vi "S4GUI.vi"(7 "Tab ObsEng":enum32{"Obs", "CCD modes", "Guider", "Eng"}(tab)) -> ()   [LabVIEW 2018] (continued)
            n4422 = call-dynamic "Write State Machine.vi"("error in (no error)"=w10331, "State Machine.lvclass"=w10334, "Device in"=w10333) -> ("error out"=w10327:errorcluster, "Device out"=w10319:refnum<class "Channel.lvclass">)  [unwired: 7 in]
            n4423 = call-dynamic "Write Channel.vi"("error in (no error)"=w10327, "Channel.lvclass"=w10319, "Acquisition in"=w10332) -> ("error out"=w10328:errorcluster, "Acquisition out"=w10330:refnum<class "Acquisition.lvclass">)  [unwired: 7 in]
            n4424 = call-dynamic "Write AcquisitionC.vi"("error in (no error)"=w10328, "Acquisition.lvclass"=w10330, "S4ACS_GUI in"=w10329) -> ("error out"=w10341:errorcluster, "S4ACS_GUI out"=w10340:refnum<class "S4GUI.lvclass">)  [unwired: 7 in]
          }
        }
      }
      event "cooler ON 4": Value Change {
        n4425 = event-data() -> ("NewVal"=w10342:bool)  [unwired: 1 in]
        n4426 = case shown="True" w10342 {
          tunnel: [w10347 w10382] -> w10346
          tunnel: [w10348 w10381] -> w10345
          tunnel: w10344 -> [w10348 w10352]
          tunnel: w10343 -> [w10347 w10351]
          frame False {
          }
          frame True {
            w10350 = i16 1 items=["Cooler OFF", "Cooler ON"] ("Cooler ON/OFF")
            n4427 = Concatenate Strings("SET COOLER " ("User Event"), "ON ", "CLICKED - CH4" ("User Event")) -> (w10354:string)
            n4428 = call-dynamic "Write User Event.vi"("error in (no error)"=w10351, "User Event"=w10354, "S4GUI in"=w10352) -> ("error out"=w10355:errorcluster, "S4GUI out"=w10357:refnum<class "S4GUI.lvclass">)  [unwired: 7 in]
            n4429 = call-dynamic "Read AcquisitionD.vi"("error in (no error)"=w10355, "S4ACS_GUI in"=w10357) -> ("error out"=w10379:errorcluster, "Acquisition.lvclass"=w10380:refnum<class "Acquisition.lvclass">, "S4ACS_GUI out"=w10370:refnum<class "S4GUI.lvclass">)  [unwired: 7 in]
            n4430 = call-dynamic "Read Channel.vi"("error in (no error)"=w10379, "Acquisition in"=w10380) -> ("error out"=w10363:errorcluster, "Channel.lvclass"=w10367:refnum<class "Channel.lvclass">, "Acquisition out"=w10373:refnum<class "Acquisition.lvclass">)  [unwired: 7 in]
            n4431 = call-dynamic "Read Interface.vi"("error in (no error)"=w10363, "Channel in"=w10367) -> ("error out"=w10358:errorcluster, "Interface.lvclass"=w10359:refnum<class "Interface.lvclass">, "Channel out"=w10366:refnum<class "Channel.lvclass">)  [unwired: 7 in]
            n4432 = call-dynamic "Write Cooler ON_OFF.vi"("error in (no error)"=w10358, "Cooler ON/OFF"=w10350, "Interface in"=w10359) -> ("error out"=w10362:errorcluster, "Interface out"=w10364:refnum<class "Interface.lvclass">)  [unwired: 7 in]
            n4433 = call-dynamic "Write Interface.vi"("error in (no error)"=w10362, "Interface.lvclass"=w10364, "Channel in"=w10366) -> ("error out"=w10361:errorcluster, "Channel out"=w10365:refnum<class "Channel.lvclass">)  [unwired: 7 in]
            n4434 = call-dynamic "Read State Machine.vi"("error in (no error)"=w10361, "Device in"=w10365) -> ("error out"=w10377:errorcluster, "State Machine.lvclass"=w10378:refnum<class "State Machine.lvclass">, "Device out"=w10374:refnum<class "Channel.lvclass">)  [unwired: 7 in]
            n4435 = call "Next State.vi"("error in (no error)"=w10377, "New_State"=u32 30, "State Machine in"=w10378) -> ("error out"=w10372:errorcluster, "State Machine out"=w10375:refnum<class "State Machine.lvclass">)  [unwired: 7 in]
            n4436 = call-dynamic "Write State Machine.vi"("error in (no error)"=w10372, "State Machine.lvclass"=w10375, "Device in"=w10374) -> ("error out"=w10368:errorcluster, "Device out"=w10360:refnum<class "Channel.lvclass">)  [unwired: 7 in]
            n4437 = call-dynamic "Write Channel.vi"("error in (no error)"=w10368, "Channel.lvclass"=w10360, "Acquisition in"=w10373) -> ("error out"=w10369:errorcluster, "Acquisition out"=w10371:refnum<class "Acquisition.lvclass">)  [unwired: 7 in]
            n4438 = call-dynamic "Write AcquisitionD.vi"("error in (no error)"=w10369, "Acquisition.lvclass"=w10371, "S4ACS_GUI in"=w10370) -> ("error out"=w10382:errorcluster, "S4ACS_GUI out"=w10381:refnum<class "S4GUI.lvclass">)  [unwired: 7 in]
          }
        }
      }
      event "cooler OFF 1": Value Change {
        n4439 = event-data() -> ("NewVal"=w10383:bool)  [unwired: 1 in]
        n4440 = case shown="True" w10383 {
          tunnel: [w10388 w10423] -> w10387
          tunnel: [w10389 w10422] -> w10386
          tunnel: w10385 -> [w10389 w10393]
          tunnel: w10384 -> [w10388 w10392]
          frame False {
          }
          frame True {
            w10391 = i16 0 items=["Cooler OFF", "Cooler ON"] ("Cooler ON/OFF")
            n4441 = Concatenate Strings("SET COOLER " ("User Event"), "OFF ", "CLICKED - CH1" ("User Event")) -> (w10395:string)
            n4442 = call-dynamic "Write User Event.vi"("error in (no error)"=w10392, "User Event"=w10395, "S4GUI in"=w10393) -> ("error out"=w10396:errorcluster, "S4GUI out"=w10398:refnum<class "S4GUI.lvclass">)  [unwired: 7 in]
            n4443 = call-dynamic "Read AcquisitionA.vi"("error in (no error)"=w10396, "S4ACS_GUI in"=w10398) -> ("error out"=w10420:errorcluster, "Acquisition.lvclass"=w10421:refnum<class "Acquisition.lvclass">, "S4ACS_GUI out"=w10411:refnum<class "S4GUI.lvclass">)  [unwired: 7 in]
            n4444 = call-dynamic "Read Channel.vi"("error in (no error)"=w10420, "Acquisition in"=w10421) -> ("error out"=w10404:errorcluster, "Channel.lvclass"=w10408:refnum<class "Channel.lvclass">, "Acquisition out"=w10414:refnum<class "Acquisition.lvclass">)  [unwired: 7 in]
            n4445 = call-dynamic "Read Interface.vi"("error in (no error)"=w10404, "Channel in"=w10408) -> ("error out"=w10399:errorcluster, "Interface.lvclass"=w10400:refnum<class "Interface.lvclass">, "Channel out"=w10407:refnum<class "Channel.lvclass">)  [unwired: 7 in]
            n4446 = call-dynamic "Write Cooler ON_OFF.vi"("error in (no error)"=w10399, "Cooler ON/OFF"=w10391, "Interface in"=w10400) -> ("error out"=w10403:errorcluster, "Interface out"=w10405:refnum<class "Interface.lvclass">)  [unwired: 7 in]
            n4447 = call-dynamic "Write Interface.vi"("error in (no error)"=w10403, "Interface.lvclass"=w10405, "Channel in"=w10407) -> ("error out"=w10402:errorcluster, "Channel out"=w10406:refnum<class "Channel.lvclass">)  [unwired: 7 in]
            n4448 = call-dynamic "Read State Machine.vi"("error in (no error)"=w10402, "Device in"=w10406) -> ("error out"=w10418:errorcluster, "State Machine.lvclass"=w10419:refnum<class "State Machine.lvclass">, "Device out"=w10415:refnum<class "Channel.lvclass">)  [unwired: 7 in]
            n4449 = call "Next State.vi"("error in (no error)"=w10418, "New_State"=u32 30, "State Machine in"=w10419) -> ("error out"=w10413:errorcluster, "State Machine out"=w10416:refnum<class "State Machine.lvclass">)  [unwired: 7 in]
            n4450 = call-dynamic "Write State Machine.vi"("error in (no error)"=w10413, "State Machine.lvclass"=w10416, "Device in"=w10415) -> ("error out"=w10409:errorcluster, "Device out"=w10401:refnum<class "Channel.lvclass">)  [unwired: 7 in]
            n4451 = call-dynamic "Write Channel.vi"("error in (no error)"=w10409, "Channel.lvclass"=w10401, "Acquisition in"=w10414) -> ("error out"=w10410:errorcluster, "Acquisition out"=w10412:refnum<class "Acquisition.lvclass">)  [unwired: 7 in]
            n4452 = call-dynamic "Write AcquisitionA.vi"("error in (no error)"=w10410, "Acquisition.lvclass"=w10412, "S4ACS_GUI in"=w10411) -> ("error out"=w10423:errorcluster, "S4ACS_GUI out"=w10422:refnum<class "S4GUI.lvclass">)  [unwired: 7 in]
          }
        }
      }
      event "cooler OFF 2": Value Change {
        n4453 = event-data() -> ("NewVal"=w10424:bool)  [unwired: 1 in]
        n4454 = case shown="True" w10424 {
          tunnel: [w10429 w10464] -> w10428
          tunnel: [w10430 w10463] -> w10427
          tunnel: w10426 -> [w10430 w10434]
          tunnel: w10425 -> [w10429 w10433]
          frame False {
          }
          frame True {
            w10432 = i16 0 items=["Cooler OFF", "Cooler ON"] ("Cooler ON/OFF")
            n4455 = Concatenate Strings("SET COOLER " ("User Event"), "OFF ", "CLICKED - CH2" ("User Event")) -> (w10436:string)
            n4456 = call-dynamic "Write User Event.vi"("error in (no error)"=w10433, "User Event"=w10436, "S4GUI in"=w10434) -> ("error out"=w10437:errorcluster, "S4GUI out"=w10439:refnum<class "S4GUI.lvclass">)  [unwired: 7 in]
            n4457 = call "Read AcquisitionB.vi"("error in (no error)"=w10437, "S4ACS_GUI in"=w10439) -> ("error out"=w10461:errorcluster, "Acquisition.lvclass"=w10462:refnum<class "Acquisition.lvclass">, "S4ACS_GUI out"=w10452:refnum<class "S4GUI.lvclass">)  [unwired: 7 in]
            n4458 = call-dynamic "Read Channel.vi"("error in (no error)"=w10461, "Acquisition in"=w10462) -> ("error out"=w10445:errorcluster, "Channel.lvclass"=w10449:refnum<class "Channel.lvclass">, "Acquisition out"=w10455:refnum<class "Acquisition.lvclass">)  [unwired: 7 in]
            n4459 = call-dynamic "Read Interface.vi"("error in (no error)"=w10445, "Channel in"=w10449) -> ("error out"=w10440:errorcluster, "Interface.lvclass"=w10441:refnum<class "Interface.lvclass">, "Channel out"=w10448:refnum<class "Channel.lvclass">)  [unwired: 7 in]
            n4460 = call-dynamic "Write Cooler ON_OFF.vi"("error in (no error)"=w10440, "Cooler ON/OFF"=w10432, "Interface in"=w10441) -> ("error out"=w10444:errorcluster, "Interface out"=w10446:refnum<class "Interface.lvclass">)  [unwired: 7 in]
            n4461 = call-dynamic "Write Interface.vi"("error in (no error)"=w10444, "Interface.lvclass"=w10446, "Channel in"=w10448) -> ("error out"=w10443:errorcluster, "Channel out"=w10447:refnum<class "Channel.lvclass">)  [unwired: 7 in]
            n4462 = call-dynamic "Read State Machine.vi"("error in (no error)"=w10443, "Device in"=w10447) -> ("error out"=w10459:errorcluster, "State Machine.lvclass"=w10460:refnum<class "State Machine.lvclass">, "Device out"=w10456:refnum<class "Channel.lvclass">)  [unwired: 7 in]
            n4463 = call "Next State.vi"("error in (no error)"=w10459, "New_State"=u32 30, "State Machine in"=w10460) -> ("error out"=w10454:errorcluster, "State Machine out"=w10457:refnum<class "State Machine.lvclass">)  [unwired: 7 in]
            n4464 = call-dynamic "Write State Machine.vi"("error in (no error)"=w10454, "State Machine.lvclass"=w10457, "Device in"=w10456) -> ("error out"=w10450:errorcluster, "Device out"=w10442:refnum<class "Channel.lvclass">)  [unwired: 7 in]
            n4465 = call-dynamic "Write Channel.vi"("error in (no error)"=w10450, "Channel.lvclass"=w10442, "Acquisition in"=w10455) -> ("error out"=w10451:errorcluster, "Acquisition out"=w10453:refnum<class "Acquisition.lvclass">)  [unwired: 7 in]
            n4466 = call "Write AcquisitionB.vi"("error in (no error)"=w10451, "Acquisition.lvclass"=w10453, "S4ACS_GUI in"=w10452) -> ("error out"=w10464:errorcluster, "S4ACS_GUI out"=w10463:refnum<class "S4GUI.lvclass">)  [unwired: 7 in]
          }
        }
      }
      event "cooler OFF 3": Value Change {
        n4467 = event-data() -> ("NewVal"=w10465:bool)  [unwired: 1 in]
        n4468 = case shown="True" w10465 {
          tunnel: [w10470 w10505] -> w10469
          tunnel: [w10471 w10504] -> w10468
          tunnel: w10467 -> [w10471 w10475]
          tunnel: w10466 -> [w10470 w10474]
          frame False {
          }
          frame True {
            w10473 = i16 0 items=["Cooler OFF", "Cooler ON"] ("Cooler ON/OFF")
            n4469 = Concatenate Strings("SET COOLER " ("User Event"), "OFF ", "CLICKED - CH3" ("User Event")) -> (w10477:string)
            n4470 = call-dynamic "Write User Event.vi"("error in (no error)"=w10474, "User Event"=w10477, "S4GUI in"=w10475) -> ("error out"=w10478:errorcluster, "S4GUI out"=w10480:refnum<class "S4GUI.lvclass">)  [unwired: 7 in]
            n4471 = call-dynamic "Read AcquisitionC.vi"("error in (no error)"=w10478, "S4ACS_GUI in"=w10480) -> ("error out"=w10502:errorcluster, "Acquisition.lvclass"=w10503:refnum<class "Acquisition.lvclass">, "S4ACS_GUI out"=w10493:refnum<class "S4GUI.lvclass">)  [unwired: 7 in]
            n4472 = call-dynamic "Read Channel.vi"("error in (no error)"=w10502, "Acquisition in"=w10503) -> ("error out"=w10486:errorcluster, "Channel.lvclass"=w10490:refnum<class "Channel.lvclass">, "Acquisition out"=w10496:refnum<class "Acquisition.lvclass">)  [unwired: 7 in]
            n4473 = call-dynamic "Read Interface.vi"("error in (no error)"=w10486, "Channel in"=w10490) -> ("error out"=w10481:errorcluster, "Interface.lvclass"=w10482:refnum<class "Interface.lvclass">, "Channel out"=w10489:refnum<class "Channel.lvclass">)  [unwired: 7 in]
            n4474 = call-dynamic "Write Cooler ON_OFF.vi"("error in (no error)"=w10481, "Cooler ON/OFF"=w10473, "Interface in"=w10482) -> ("error out"=w10485:errorcluster, "Interface out"=w10487:refnum<class "Interface.lvclass">)  [unwired: 7 in]
            n4475 = call-dynamic "Write Interface.vi"("error in (no error)"=w10485, "Interface.lvclass"=w10487, "Channel in"=w10489) -> ("error out"=w10484:errorcluster, "Channel out"=w10488:refnum<class "Channel.lvclass">)  [unwired: 7 in]
            n4476 = call-dynamic "Read State Machine.vi"("error in (no error)"=w10484, "Device in"=w10488) -> ("error out"=w10500:errorcluster, "State Machine.lvclass"=w10501:refnum<class "State Machine.lvclass">, "Device out"=w10497:refnum<class "Channel.lvclass">)  [unwired: 7 in]
            n4477 = call "Next State.vi"("error in (no error)"=w10500, "New_State"=u32 30, "State Machine in"=w10501) -> ("error out"=w10495:errorcluster, "State Machine out"=w10498:refnum<class "State Machine.lvclass">)  [unwired: 7 in]
            n4478 = call-dynamic "Write State Machine.vi"("error in (no error)"=w10495, "State Machine.lvclass"=w10498, "Device in"=w10497) -> ("error out"=w10491:errorcluster, "Device out"=w10483:refnum<class "Channel.lvclass">)  [unwired: 7 in]
            n4479 = call-dynamic "Write Channel.vi"("error in (no error)"=w10491, "Channel.lvclass"=w10483, "Acquisition in"=w10496) -> ("error out"=w10492:errorcluster, "Acquisition out"=w10494:refnum<class "Acquisition.lvclass">)  [unwired: 7 in]
            n4480 = call-dynamic "Write AcquisitionC.vi"("error in (no error)"=w10492, "Acquisition.lvclass"=w10494, "S4ACS_GUI in"=w10493) -> ("error out"=w10505:errorcluster, "S4ACS_GUI out"=w10504:refnum<class "S4GUI.lvclass">)  [unwired: 7 in]
          }
        }
      }
      event "cooler OFF 4": Value Change {
        n4481 = event-data() -> ("NewVal"=w10506:bool)  [unwired: 1 in]
        n4482 = case shown="True" w10506 {
          tunnel: [w10511 w10546] -> w10510
          tunnel: [w10512 w10545] -> w10509
          tunnel: w10508 -> [w10512 w10516]
          tunnel: w10507 -> [w10511 w10515]
          frame False {
          }
          frame True {
            w10514 = i16 0 items=["Cooler OFF", "Cooler ON"] ("Cooler ON/OFF")
            n4483 = Concatenate Strings("SET COOLER " ("User Event"), "OFF ", "CLICKED - CH4" ("User Event")) -> (w10518:string)
            n4484 = call-dynamic "Write User Event.vi"("error in (no error)"=w10515, "User Event"=w10518, "S4GUI in"=w10516) -> ("error out"=w10519:errorcluster, "S4GUI out"=w10521:refnum<class "S4GUI.lvclass">)  [unwired: 7 in]
            n4485 = call-dynamic "Read AcquisitionD.vi"("error in (no error)"=w10519, "S4ACS_GUI in"=w10521) -> ("error out"=w10543:errorcluster, "Acquisition.lvclass"=w10544:refnum<class "Acquisition.lvclass">, "S4ACS_GUI out"=w10534:refnum<class "S4GUI.lvclass">)  [unwired: 7 in]
            n4486 = call-dynamic "Read Channel.vi"("error in (no error)"=w10543, "Acquisition in"=w10544) -> ("error out"=w10527:errorcluster, "Channel.lvclass"=w10531:refnum<class "Channel.lvclass">, "Acquisition out"=w10537:refnum<class "Acquisition.lvclass">)  [unwired: 7 in]
            n4487 = call-dynamic "Read Interface.vi"("error in (no error)"=w10527, "Channel in"=w10531) -> ("error out"=w10522:errorcluster, "Interface.lvclass"=w10523:refnum<class "Interface.lvclass">, "Channel out"=w10530:refnum<class "Channel.lvclass">)  [unwired: 7 in]
            n4488 = call-dynamic "Write Cooler ON_OFF.vi"("error in (no error)"=w10522, "Cooler ON/OFF"=w10514, "Interface in"=w10523) -> ("error out"=w10526:errorcluster, "Interface out"=w10528:refnum<class "Interface.lvclass">)  [unwired: 7 in]
            n4489 = call-dynamic "Write Interface.vi"("error in (no error)"=w10526, "Interface.lvclass"=w10528, "Channel in"=w10530) -> ("error out"=w10525:errorcluster, "Channel out"=w10529:refnum<class "Channel.lvclass">)  [unwired: 7 in]
            n4490 = call-dynamic "Read State Machine.vi"("error in (no error)"=w10525, "Device in"=w10529) -> ("error out"=w10541:errorcluster, "State Machine.lvclass"=w10542:refnum<class "State Machine.lvclass">, "Device out"=w10538:refnum<class "Channel.lvclass">)  [unwired: 7 in]
            n4491 = call "Next State.vi"("error in (no error)"=w10541, "New_State"=u32 30, "State Machine in"=w10542) -> ("error out"=w10536:errorcluster, "State Machine out"=w10539:refnum<class "State Machine.lvclass">)  [unwired: 7 in]
            n4492 = call-dynamic "Write State Machine.vi"("error in (no error)"=w10536, "State Machine.lvclass"=w10539, "Device in"=w10538) -> ("error out"=w10532:errorcluster, "Device out"=w10524:refnum<class "Channel.lvclass">)  [unwired: 7 in]
            n4493 = call-dynamic "Write Channel.vi"("error in (no error)"=w10532, "Channel.lvclass"=w10524, "Acquisition in"=w10537) -> ("error out"=w10533:errorcluster, "Acquisition out"=w10535:refnum<class "Acquisition.lvclass">)  [unwired: 7 in]
            n4494 = call-dynamic "Write AcquisitionD.vi"("error in (no error)"=w10533, "Acquisition.lvclass"=w10535, "S4ACS_GUI in"=w10534) -> ("error out"=w10546:errorcluster, "S4ACS_GUI out"=w10545:refnum<class "S4GUI.lvclass">)  [unwired: 7 in]
          }
        }
      }
      event "Set Temp 1": Value Change {
        n4495 = event-data() -> ("NewVal"=w10547:bool)  [unwired: 1 in]
        n4496 = case shown="True" w10547 {
          tunnel: w10551 -> [w10553 w10570]
          tunnel: w10550 -> [w10552 w10569]
          tunnel: [w10552 w10559] -> w10549
          tunnel: [w10553 w10560] -> w10548
          frame False {
          }
          frame True {
            # "Carrega a maior temperatura\nentre target atual e o target do controle."
            # "Carrega o valor da temperatura target de acordo com a conf CCD"
            n4497 = call-dynamic "Read AcquisitionA.vi"("error in (no error)"=w10569, "S4ACS_GUI in"=w10570) -> ("error out"=w10572:errorcluster, "Acquisition.lvclass"=w10571:refnum<class "Acquisition.lvclass">, "S4ACS_GUI out"=w10556:refnum<class "S4GUI.lvclass">)  [unwired: 7 in]
            n4498 = call-dynamic "Read Channel.vi"("error in (no error)"=w10572, "Acquisition in"=w10571) -> ("error out"=w10583:errorcluster, "Channel.lvclass"=w10582:refnum<class "Channel.lvclass">, "Acquisition out"=w10555:refnum<class "Acquisition.lvclass">)  [unwired: 7 in]
            n4499 = call-dynamic "ValidateConfig.vi"("error in (no error)"=w10583, "Channel in"=w10582) -> ("error out"=w10589:errorcluster, "Channel out"=w10588:refnum<class "Channel.lvclass">)  [unwired: 7 in, 1 out]
            n4500 = call-dynamic "Read Interface.vi"("error in (no error)"=w10589, "Channel in"=w10588) -> ("error out"=w10585:errorcluster, "Interface.lvclass"=w10584:refnum<class "Interface.lvclass">, "Channel out"=w10578:refnum<class "Channel.lvclass">)  [unwired: 7 in]
            n4501 = call-dynamic "Read Temperature.vi"("error in (no error)"=w10585, "Interface in"=w10584) -> ("error out"=w10586:errorcluster, "Temperature"=w10590:i8, "Interface out"=w10587:refnum<class "Interface.lvclass">)  [unwired: 7 in]
            n4502 = Greater?(x=w10590, y="Target Temp 1") -> (0:w10558:bool)
            n4503 = Select(t=w10590, s=w10558, f="Target Temp 1") -> (s? t:f=w10563:i8)
            n4504 = call-dynamic "Write Temperature.vi"("error in (no error)"=w10586, "Temperature"=w10563, "Interface in"=w10587) -> ("error out"=w10580:errorcluster, "Interface out"=w10577:refnum<class "Interface.lvclass">)  [unwired: 7 in]
            n4505 = call-dynamic "Write Interface.vi"("error in (no error)"=w10580, "Interface.lvclass"=w10577, "Channel in"=w10578) -> ("error out"=w10581:errorcluster, "Channel out"=w10579:refnum<class "Channel.lvclass">)  [unwired: 7 in]
            n4506 = case shown="True" w10558 {
              tunnel: w10581 -> [w10615 w10618]
              tunnel: w10579 -> [w10614 w10625]
              tunnel: [w10613 w10625] -> w10576
              tunnel: [w10612 w10624] -> w10575
              tunnel: w10556 -> [w10592 w10620]
              tunnel: [w10592 w10623] -> w10557
              tunnel: w10555 -> [w10591 w10622]
              tunnel: [w10591 w10621] -> w10554
              frame False {
                # "input ok"
                n4507 = call-dynamic "Read State Machine.vi"("error in (no error)"=w10615, "Device in"=w10614) -> ("error out"=w10594:errorcluster, "State Machine.lvclass"=w10601:refnum<class "State Machine.lvclass">, "Device out"=w10610:refnum<class "Channel.lvclass">)  [unwired: 7 in]
                n4508 = call-dynamic "Read ref StatesQueue.vi"("error in (no error)"=w10594, "State Machine in"=w10601) -> ("error out"=w10604:errorcluster, "ref StatesQueue"=w10598:refnum<queue>, "State Machine out"=w10600:refnum<class "State Machine.lvclass">)  [unwired: 7 in]
                n4509 = Flush Queue(queue=w10598, error in (no error)=w10604) -> (queue out=w10597:refnum<queue>, error out=w10606:errorcluster)  [unwired: 1 out]
                n4510 = Enqueue Element(queue=w10597, element=u32 35 ("State"), error in (no error)=w10606) -> (queue out=w10596:refnum<queue>, error out=w10607:errorcluster)  [unwired: 1 in, 1 out]
                n4511 = Enqueue Element(queue=w10596, element=u32 37 ("State"), error in (no error)=w10607) -> (queue out=w10595:refnum<queue>, error out=w10605:errorcluster)  [unwired: 1 in, 1 out]
                n4512 = call-dynamic "Write ref StatesQueue.vi"("error in (no error)"=w10605, "ref StatesQueue"=w10595, "State Machine in"=w10600) -> ("error out"=w10593:errorcluster, "State Machine out"=w10599:refnum<class "State Machine.lvclass">)  [unwired: 7 in]
                n4513 = call "Next State.vi"("error in (no error)"=w10593, "New_State"=u32 0, "State Machine in"=w10599) -> ("error out"=w10611:errorcluster, "State Machine out"=w10609:refnum<class "State Machine.lvclass">)  [unwired: 7 in]
                n4514 = call-dynamic "Write State Machine.vi"("error in (no error)"=w10611, "State Machine.lvclass"=w10609, "Device in"=w10610) -> ("error out"=w10612:errorcluster, "Device out"=w10613:refnum<class "Channel.lvclass">)  [unwired: 7 in]
              }
              frame True {
                # "input error"
                n4515 = call-dynamic "Read SET temp error mode.vi"("error in (no error)"=w10618, "S4GUI in"=w10620) -> ("error out"=w10617:errorcluster, "SET temp error mode"=w10616:bool, "S4GUI out"=w10619:refnum<class "S4GUI.lvclass">)  [unwired: 7 in]
                n4516 = case shown="False" w10616 {
                  tunnel: [w10634 w10649] -> w10624
                  tunnel: [w10633 w10648] -> w10623
                  tunnel: w10619 -> [w10632 w10648]
                  tunnel: w10617 -> [w10629 w10650]
                  tunnel: w10622 -> [w10627 w10647]
                  tunnel: [w10626 w10647] -> w10621
                  frame False {
                    # "last error msg"
                    n4517 = call-dynamic "Read sync.vi"("error in (no error)"=w10629, "S4ACS_GUI in"=w10632) -> ("error out"=w10628:errorcluster, "sync"=w10630:bool, "S4ACS_GUI out"=w10631:refnum<class "S4GUI.lvclass">)  [unwired: 7 in]
                    n4518 = case shown="False" w10630 {
                      tunnel: w10628 -> [w10637 w10646]
                      tunnel: [w10636 w10645] -> w10634
                      tunnel: [w10640 w10644] -> w10633
                      tunnel: w10631 -> [w10640 w10642]
                      tunnel: w10627 -> [w10638 w10641]
                      tunnel: [w10635 w10641] -> w10626
                      frame False {
                        n4519 = call-dynamic "Write Acq_state.vi"("error in (no error)"=w10637, "Acq_state"=u32 240, "Acquisition in"=w10638) -> ("error out"=w10636:errorcluster, "Acquisition out"=w10635:refnum<class "Acquisition.lvclass">)  [unwired: 7 in]
                      }
                      frame True {
                        n4520 = call-dynamic "Write Obs_state.vi"("error in (no error)"=w10646, "Obs_state"=u32 240, "S4ACS_GUI in"=w10642) -> ("error out"=w10645:errorcluster, "S4ACS_GUI out"=w10644:refnum<class "S4GUI.lvclass">)  [unwired: 7 in]
                      }
                    }
                  }
                  frame True {
                    # "popup msg"
                    n4521 = disable-structure shown="Enabled" {
                      disable-tunnel: w10650 -> [w10652 w10659]
                      disable-tunnel: [w10651 w10659] -> w10649
                      frame Enabled {
                        w10654 = FALSE ("Wait Until Done")
                        n4522 = call <vilib>:"Application Directory.vi"() -> ("Application Directory"=w10658:path)
                        n4523 = Build Path(base path=w10658, name or relative path="MsgSetTemp.vi") -> (appended path=w10655:path)
                        n4524 = Open VI Reference(vi path=w10655, error in (no error)=w10652) -> (vi reference=w10656:refnum<vi>, error out=w10657:errorcluster)  [unwired: 4 in]
                        n4525 = invoke class="VI" method="Run VI"(reference=w10656, error in=w10657, "Wait until done"=w10654, "Auto Dispose Ref"=w10654) -> (error out=w10651:errorcluster)  [unwired: 1 in, 4 out]
                      }
                      frame Disabled {
                        n4526 = One Button Dialog(message="ERROR: Invalid input value. It must be \nequal or greater than the minimum for \nthe current CCD setup.", button name ("OK")="OK" ("T button name (\"OK\")")) -> ()  [unwired: 1 out]
                      }
                    }
                  }
                }
              }
            }
            n4527 = Number To Decimal String(number="Target Temp 1") -> (decimal integer string=w10562:string)  [unwired: 1 in]
            n4528 = call-dynamic "Write Channel.vi"("error in (no error)"=w10575, "Channel.lvclass"=w10576, "Acquisition in"=w10554) -> ("error out"=w10574:errorcluster, "Acquisition out"=w10573:refnum<class "Acquisition.lvclass">)  [unwired: 7 in]
            n4529 = Concatenate Strings("SET TEMP [" ("User Event"), w10562, "] CLICKED - CH1" ("User Event")) -> (w10568:string)
            n4530 = call-dynamic "Write AcquisitionA.vi"("error in (no error)"=w10574, "Acquisition.lvclass"=w10573, "S4ACS_GUI in"=w10557) -> ("error out"=w10564:errorcluster, "S4ACS_GUI out"=w10565:refnum<class "S4GUI.lvclass">)  [unwired: 7 in]
            n4531 = call-dynamic "Write User Event.vi"("error in (no error)"=w10564, "User Event"=w10568, "S4GUI in"=w10565) -> ("error out"=w10559:errorcluster, "S4GUI out"=w10560:refnum<class "S4GUI.lvclass">)  [unwired: 7 in]
          }
        }
      }
      event "Set Temp 2": Value Change {
        n4532 = event-data() -> ("NewVal"=w10662:bool)  [unwired: 1 in]
        n4533 = case shown="True" w10662 {
          tunnel: w10666 -> [w10668 w10688]
          tunnel: w10665 -> [w10667 w10687]
          tunnel: [w10667 w10680] -> w10664
          tunnel: [w10668 w10682] -> w10663
          frame False {
          }
          frame True {
            # "Carrega a maior temperatura\nentre target atual e o target do controle."
            # "Carrega o valor da temperatura target de acordo com a conf CCD"
            n4534 = call "Read AcquisitionB.vi"("error in (no error)"=w10687, "S4ACS_GUI in"=w10688) -> ("error out"=w10704:errorcluster, "Acquisition.lvclass"=w10705:refnum<class "Acquisition.lvclass">, "S4ACS_GUI out"=w10675:refnum<class "S4GUI.lvclass">)  [unwired: 7 in]
            n4535 = call-dynamic "Read Channel.vi"("error in (no error)"=w10704, "Acquisition in"=w10705) -> ("error out"=w10697:errorcluster, "Channel.lvclass"=w10698:refnum<class "Channel.lvclass">, "Acquisition out"=w10676:refnum<class "Acquisition.lvclass">)  [unwired: 7 in]
            n4536 = call-dynamic "ValidateConfig.vi"("error in (no error)"=w10697, "Channel in"=w10698) -> ("error out"=w10691:errorcluster, "Channel out"=w10692:refnum<class "Channel.lvclass">)  [unwired: 7 in, 1 out]
            n4537 = call-dynamic "Read Interface.vi"("error in (no error)"=w10691, "Channel in"=w10692) -> ("error out"=w10695:errorcluster, "Interface.lvclass"=w10696:refnum<class "Interface.lvclass">, "Channel out"=w10700:refnum<class "Channel.lvclass">)  [unwired: 7 in]
            n4538 = call-dynamic "Read Temperature.vi"("error in (no error)"=w10695, "Interface in"=w10696) -> ("error out"=w10694:errorcluster, "Temperature"=w10690:i8, "Interface out"=w10693:refnum<class "Interface.lvclass">)  [unwired: 7 in]
            n4539 = Greater?(x=w10690, y="Target Temp 2") -> (0:w10673:bool)
            n4540 = Select(t=w10690, s=w10673, f="Target Temp 2") -> (s? t:f=w10689:i32)
            n4541 = call-dynamic "Write Temperature.vi"("error in (no error)"=w10694, "Temperature"=w10689, "Interface in"=w10693) -> ("error out"=w10699:errorcluster, "Interface out"=w10701:refnum<class "Interface.lvclass">)  [unwired: 7 in]
            n4542 = call-dynamic "Write Interface.vi"("error in (no error)"=w10699, "Interface.lvclass"=w10701, "Channel in"=w10700) -> ("error out"=w10674:errorcluster, "Channel out"=w10677:refnum<class "Channel.lvclass">)  [unwired: 7 in]
            n4543 = case shown="True" w10673 {
              tunnel: w10674 -> [w10730 w10735]
              tunnel: w10677 -> [w10729 w10737]
              tunnel: [w10728 w10737] -> w10670
              tunnel: [w10727 w10740] -> w10669
              tunnel: w10675 -> [w10707 w10736]
              tunnel: [w10707 w10739] -> w10672
              tunnel: w10676 -> [w10706 w10731]
              tunnel: [w10706 w10738] -> w10671
              frame False {
                # "input ok"
                n4544 = call-dynamic "Read State Machine.vi"("error in (no error)"=w10730, "Device in"=w10729) -> ("error out"=w10709:errorcluster, "State Machine.lvclass"=w10716:refnum<class "State Machine.lvclass">, "Device out"=w10725:refnum<class "Channel.lvclass">)  [unwired: 7 in]
                n4545 = call-dynamic "Read ref StatesQueue.vi"("error in (no error)"=w10709, "State Machine in"=w10716) -> ("error out"=w10719:errorcluster, "ref StatesQueue"=w10713:refnum<queue>, "State Machine out"=w10715:refnum<class "State Machine.lvclass">)  [unwired: 7 in]
                n4546 = Flush Queue(queue=w10713, error in (no error)=w10719) -> (queue out=w10712:refnum<queue>, error out=w10721:errorcluster)  [unwired: 1 out]
                n4547 = Enqueue Element(queue=w10712, element=u32 35 ("State"), error in (no error)=w10721) -> (queue out=w10711:refnum<queue>, error out=w10722:errorcluster)  [unwired: 1 in, 1 out]
                n4548 = Enqueue Element(queue=w10711, element=u32 37 ("State"), error in (no error)=w10722) -> (queue out=w10710:refnum<queue>, error out=w10720:errorcluster)  [unwired: 1 in, 1 out]
                n4549 = call-dynamic "Write ref StatesQueue.vi"("error in (no error)"=w10720, "ref StatesQueue"=w10710, "State Machine in"=w10715) -> ("error out"=w10708:errorcluster, "State Machine out"=w10714:refnum<class "State Machine.lvclass">)  [unwired: 7 in]
                n4550 = call "Next State.vi"("error in (no error)"=w10708, "New_State"=u32 0, "State Machine in"=w10714) -> ("error out"=w10726:errorcluster, "State Machine out"=w10724:refnum<class "State Machine.lvclass">)  [unwired: 7 in]
                n4551 = call-dynamic "Write State Machine.vi"("error in (no error)"=w10726, "State Machine.lvclass"=w10724, "Device in"=w10725) -> ("error out"=w10727:errorcluster, "Device out"=w10728:refnum<class "Channel.lvclass">)  [unwired: 7 in]
              }
              frame True {
                # "input error"
                n4552 = call-dynamic "Read SET temp error mode.vi"("error in (no error)"=w10735, "S4GUI in"=w10736) -> ("error out"=w10732:errorcluster, "SET temp error mode"=w10734:bool, "S4GUI out"=w10733:refnum<class "S4GUI.lvclass">)  [unwired: 7 in]
                n4553 = case shown="False" w10734 {
                  tunnel: [w10749 w10762] -> w10740
                  tunnel: [w10748 w10771] -> w10739
                  tunnel: [w10744 w10770] -> w10738
                  tunnel: w10731 -> [w10743 w10770]
                  tunnel: w10733 -> [w10742 w10771]
                  tunnel: w10732 -> [w10741 w10763]
                  frame False {
                    # "last error msg"
                    n4554 = call-dynamic "Read sync.vi"("error in (no error)"=w10741, "S4ACS_GUI in"=w10742) -> ("error out"=w10745:errorcluster, "sync"=w10746:bool, "S4ACS_GUI out"=w10747:refnum<class "S4GUI.lvclass">)  [unwired: 7 in]
                    n4555 = case shown="True" w10746 {
                      tunnel: w10745 -> [w10752 w10761]
                      tunnel: [w10751 w10760] -> w10749
                      tunnel: [w10755 w10759] -> w10748
                      tunnel: w10747 -> [w10755 w10757]
                      tunnel: w10743 -> [w10753 w10756]
                      tunnel: [w10750 w10756] -> w10744
                      frame False {
                        n4556 = call-dynamic "Write Acq_state.vi"("error in (no error)"=w10752, "Acq_state"=u32 240, "Acquisition in"=w10753) -> ("error out"=w10751:errorcluster, "Acquisition out"=w10750:refnum<class "Acquisition.lvclass">)  [unwired: 7 in]
                      }
                      frame True {
                        n4557 = call-dynamic "Write Obs_state.vi"("error in (no error)"=w10761, "Obs_state"=u32 240, "S4ACS_GUI in"=w10757) -> ("error out"=w10760:errorcluster, "S4ACS_GUI out"=w10759:refnum<class "S4GUI.lvclass">)  [unwired: 7 in]
                      }
                    }
                  }
                  frame True {
                    w10765 = FALSE ("Wait Until Done")
                    # "popup msg"
                    n4558 = call <vilib>:"Application Directory.vi"() -> ("Application Directory"=w10769:path)
                    n4559 = Build Path(base path=w10769, name or relative path="MsgSetTemp.vi") -> (appended path=w10766:path)
                    n4560 = Open VI Reference(vi path=w10766, error in (no error)=w10763) -> (vi reference=w10767:refnum<vi>, error out=w10768:errorcluster)  [unwired: 4 in]
                    n4561 = invoke class="VI" method="Run VI"(reference=w10767, error in=w10768, "Wait until done"=w10765, "Auto Dispose Ref"=w10765) -> (error out=w10762:errorcluster)  [unwired: 1 in, 4 out]
                  }
                }
              }
            }
            n4562 = Number To Decimal String(number="Target Temp 2") -> (decimal integer string=w10678:string)  [unwired: 1 in]
            n4563 = call-dynamic "Write Channel.vi"("error in (no error)"=w10669, "Channel.lvclass"=w10670, "Acquisition in"=w10671) -> ("error out"=w10702:errorcluster, "Acquisition out"=w10703:refnum<class "Acquisition.lvclass">)  [unwired: 7 in]
            n4564 = Concatenate Strings("SET TEMP [" ("User Event"), w10678, "] CLICKED - CH2" ("User Event")) -> (w10686:string)
            n4565 = call "Write AcquisitionB.vi"("error in (no error)"=w10702, "Acquisition.lvclass"=w10703, "S4ACS_GUI in"=w10672) -> ("error out"=w10681:errorcluster, "S4ACS_GUI out"=w10683:refnum<class "S4GUI.lvclass">)  [unwired: 7 in]
            n4566 = call-dynamic "Write User Event.vi"("error in (no error)"=w10681, "User Event"=w10686, "S4GUI in"=w10683) -> ("error out"=w10680:errorcluster, "S4GUI out"=w10682:refnum<class "S4GUI.lvclass">)  [unwired: 7 in]
          }
        }
      }
      event "Set Temp 3": Value Change {
        n4567 = event-data() -> ("NewVal"=w10772:bool)  [unwired: 1 in]
        n4568 = case shown="True" w10772 {
          tunnel: w10776 -> [w10778 w10798]
          tunnel: w10775 -> [w10777 w10797]
          tunnel: [w10777 w10789] -> w10774
          tunnel: [w10778 w10791] -> w10773
          frame False {
          }
          frame True {
            # "Carrega a maior temperatura\nentre target atual e o target do controle."
            # "Carrega o valor da temperatura target de acordo com a conf CCD"
            n4569 = call-dynamic "Read AcquisitionC.vi"("error in (no error)"=w10797, "S4ACS_GUI in"=w10798) -> ("error out"=w10800:errorcluster, "Acquisition.lvclass"=w10799:refnum<class "Acquisition.lvclass">, "S4ACS_GUI out"=w10780:refnum<class "S4GUI.lvclass">)  [unwired: 7 in]
            n4570 = call-dynamic "Read Channel.vi"("error in (no error)"=w10800, "Acquisition in"=w10799) -> ("error out"=w10807:errorcluster, "Channel.lvclass"=w10806:refnum<class "Channel.lvclass">, "Acquisition out"=w10781:refnum<class "Acquisition.lvclass">)  [unwired: 7 in]
            n4571 = call-dynamic "ValidateConfig.vi"("error in (no error)"=w10807, "Channel in"=w10806) -> ("error out"=w10813:errorcluster, "Channel out"=w10812:refnum<class "Channel.lvclass">)  [unwired: 7 in, 1 out]
            n4572 = call-dynamic "Read Interface.vi"("error in (no error)"=w10813, "Channel in"=w10812) -> ("error out"=w10809:errorcluster, "Interface.lvclass"=w10808:refnum<class "Interface.lvclass">, "Channel out"=w10804:refnum<class "Channel.lvclass">)  [unwired: 7 in]
            n4573 = call-dynamic "Read Temperature.vi"("error in (no error)"=w10809, "Interface in"=w10808) -> ("error out"=w10810:errorcluster, "Temperature"=w10814:i8, "Interface out"=w10811:refnum<class "Interface.lvclass">)  [unwired: 7 in]
            n4574 = Greater?(x=w10814, y="Target Temp 3") -> (0:w10779:bool)
            n4575 = Select(t=w10814, s=w10779, f="Target Temp 3") -> (s? t:f=w10815:i32)
            n4576 = call-dynamic "Write Temperature.vi"("error in (no error)"=w10810, "Temperature"=w10815, "Interface in"=w10811) -> ("error out"=w10805:errorcluster, "Interface out"=w10803:refnum<class "Interface.lvclass">)  [unwired: 7 in]
            n4577 = call-dynamic "Write Interface.vi"("error in (no error)"=w10805, "Interface.lvclass"=w10803, "Channel in"=w10804) -> ("error out"=w10782:errorcluster, "Channel out"=w10787:refnum<class "Channel.lvclass">)  [unwired: 7 in]
            n4578 = case shown="True" w10779 {
              tunnel: w10782 -> [w10840 w10841]
              tunnel: w10787 -> [w10839 w10847]
              tunnel: [w10838 w10847] -> w10786
              tunnel: [w10837 w10850] -> w10783
              tunnel: w10780 -> [w10817 w10846]
              tunnel: [w10817 w10849] -> w10784
              tunnel: w10781 -> [w10816 w10844]
              tunnel: [w10816 w10848] -> w10785
              frame False {
                # "input ok"
                n4579 = call-dynamic "Read State Machine.vi"("error in (no error)"=w10840, "Device in"=w10839) -> ("error out"=w10819:errorcluster, "State Machine.lvclass"=w10826:refnum<class "State Machine.lvclass">, "Device out"=w10835:refnum<class "Channel.lvclass">)  [unwired: 7 in]
                n4580 = call-dynamic "Read ref StatesQueue.vi"("error in (no error)"=w10819, "State Machine in"=w10826) -> ("error out"=w10829:errorcluster, "ref StatesQueue"=w10823:refnum<queue>, "State Machine out"=w10825:refnum<class "State Machine.lvclass">)  [unwired: 7 in]
                n4581 = Flush Queue(queue=w10823, error in (no error)=w10829) -> (queue out=w10822:refnum<queue>, error out=w10831:errorcluster)  [unwired: 1 out]
                n4582 = Enqueue Element(queue=w10822, element=u32 35 ("State"), error in (no error)=w10831) -> (queue out=w10821:refnum<queue>, error out=w10832:errorcluster)  [unwired: 1 in, 1 out]
                n4583 = Enqueue Element(queue=w10821, element=u32 37 ("State"), error in (no error)=w10832) -> (queue out=w10820:refnum<queue>, error out=w10830:errorcluster)  [unwired: 1 in, 1 out]
                n4584 = call-dynamic "Write ref StatesQueue.vi"("error in (no error)"=w10830, "ref StatesQueue"=w10820, "State Machine in"=w10825) -> ("error out"=w10818:errorcluster, "State Machine out"=w10824:refnum<class "State Machine.lvclass">)  [unwired: 7 in]
                n4585 = call "Next State.vi"("error in (no error)"=w10818, "New_State"=u32 0, "State Machine in"=w10824) -> ("error out"=w10836:errorcluster, "State Machine out"=w10834:refnum<class "State Machine.lvclass">)  [unwired: 7 in]
                n4586 = call-dynamic "Write State Machine.vi"("error in (no error)"=w10836, "State Machine.lvclass"=w10834, "Device in"=w10835) -> ("error out"=w10837:errorcluster, "Device out"=w10838:refnum<class "Channel.lvclass">)  [unwired: 7 in]
              }
              frame True {
                # "input error"
                n4587 = call-dynamic "Read SET temp error mode.vi"("error in (no error)"=w10841, "S4GUI in"=w10846) -> ("error out"=w10842:errorcluster, "SET temp error mode"=w10843:bool, "S4GUI out"=w10845:refnum<class "S4GUI.lvclass">)  [unwired: 7 in]
                n4588 = case shown="False" w10843 {
                  tunnel: [w10859 w10872] -> w10850
                  tunnel: [w10858 w10881] -> w10849
                  tunnel: w10845 -> [w10857 w10881]
                  tunnel: w10842 -> [w10854 w10873]
                  tunnel: w10844 -> [w10852 w10880]
                  tunnel: [w10851 w10880] -> w10848
                  frame False {
                    # "last error msg"
                    n4589 = call-dynamic "Read sync.vi"("error in (no error)"=w10854, "S4ACS_GUI in"=w10857) -> ("error out"=w10853:errorcluster, "sync"=w10855:bool, "S4ACS_GUI out"=w10856:refnum<class "S4GUI.lvclass">)  [unwired: 7 in]
                    n4590 = case shown="True" w10855 {
                      tunnel: w10853 -> [w10862 w10871]
                      tunnel: [w10861 w10870] -> w10859
                      tunnel: [w10865 w10869] -> w10858
                      tunnel: w10856 -> [w10865 w10867]
                      tunnel: w10852 -> [w10863 w10866]
                      tunnel: [w10860 w10866] -> w10851
                      frame False {
                        n4591 = call-dynamic "Write Acq_state.vi"("error in (no error)"=w10862, "Acq_state"=u32 240, "Acquisition in"=w10863) -> ("error out"=w10861:errorcluster, "Acquisition out"=w10860:refnum<class "Acquisition.lvclass">)  [unwired: 7 in]
                      }
                      frame True {
                        n4592 = call-dynamic "Write Obs_state.vi"("error in (no error)"=w10871, "Obs_state"=u32 240, "S4ACS_GUI in"=w10867) -> ("error out"=w10870:errorcluster, "S4ACS_GUI out"=w10869:refnum<class "S4GUI.lvclass">)  [unwired: 7 in]
                      }
                    }
                  }
                  frame True {
                    w10875 = FALSE ("Wait Until Done")
                    # "popup msg"
                    n4593 = call <vilib>:"Application Directory.vi"() -> ("Application Directory"=w10876:path)
                    n4594 = Build Path(base path=w10876, name or relative path="MsgSetTemp.vi") -> (appended path=w10879:path)
                    n4595 = Open VI Reference(vi path=w10879, error in (no error)=w10873) -> (vi reference=w10878:refnum<vi>, error out=w10877:errorcluster)  [unwired: 4 in]
                    n4596 = invoke class="VI" method="Run VI"(reference=w10878, error in=w10877, "Wait until done"=w10875, "Auto Dispose Ref"=w10875) -> (error out=w10872:errorcluster)  [unwired: 1 in, 4 out]
                  }
                }
              }
            }
            n4597 = Number To Decimal String(number="Target Temp 3") -> (decimal integer string=w10793:string)  [unwired: 1 in]
            n4598 = call-dynamic "Write Channel.vi"("error in (no error)"=w10783, "Channel.lvclass"=w10786, "Acquisition in"=w10785) -> ("error out"=w10802:errorcluster, "Acquisition out"=w10801:refnum<class "Acquisition.lvclass">)  [unwired: 7 in]
            n4599 = call-dynamic "Write AcquisitionC.vi"("error in (no error)"=w10802, "Acquisition.lvclass"=w10801, "S4ACS_GUI in"=w10784) -> ("error out"=w10790:errorcluster, "S4ACS_GUI out"=w10792:refnum<class "S4GUI.lvclass">)  [unwired: 7 in]
            n4600 = Concatenate Strings("SET TEMP [" ("User Event"), w10793, "] CLICKED - CH3" ("User Event")) -> (w10796:string)
            n4601 = call-dynamic "Write User Event.vi"("error in (no error)"=w10790, "User Event"=w10796, "S4GUI in"=w10792) -> ("error out"=w10789:errorcluster, "S4GUI out"=w10791:refnum<class "S4GUI.lvclass">)  [unwired: 7 in]
          }
        }
      }
      event "Set Temp 4": Value Change {
        n4602 = event-data() -> ("NewVal"=w10882:bool)  [unwired: 1 in]
        n4603 = case shown="True" w10882 {
          tunnel: w10886 -> [w10888 w10921]
          tunnel: w10885 -> [w10887 w10920]
          tunnel: [w10887 w10898] -> w10884
          tunnel: [w10888 w10899] -> w10883
          frame False {
          }
          frame True {
            # "Carrega a maior temperatura\nentre target atual e o target do controle."
            # "Carrega o valor da temperatura target de acordo com a conf CCD"
            n4604 = call-dynamic "Read AcquisitionD.vi"("error in (no error)"=w10920, "S4ACS_GUI in"=w10921) -> ("error out"=w10924:errorcluster, "Acquisition.lvclass"=w10925:refnum<class "Acquisition.lvclass">, "S4ACS_GUI out"=w10894:refnum<class "S4GUI.lvclass">)  [unwired: 7 in]
            n4605 = call-dynamic "Read Channel.vi"("error in (no error)"=w10924, "Acquisition in"=w10925) -> ("error out"=w10915:errorcluster, "Channel.lvclass"=w10916:refnum<class "Channel.lvclass">, "Acquisition out"=w10895:refnum<class "Acquisition.lvclass">)  [unwired: 7 in]
            n4606 = call-dynamic "ValidateConfig.vi"("error in (no error)"=w10915, "Channel in"=w10916) -> ("error out"=w10909:errorcluster, "Channel out"=w10910:refnum<class "Channel.lvclass">)  [unwired: 7 in, 1 out]
            n4607 = call-dynamic "Read Interface.vi"("error in (no error)"=w10909, "Channel in"=w10910) -> ("error out"=w10913:errorcluster, "Interface.lvclass"=w10914:refnum<class "Interface.lvclass">, "Channel out"=w10918:refnum<class "Channel.lvclass">)  [unwired: 7 in]
            n4608 = call-dynamic "Read Temperature.vi"("error in (no error)"=w10913, "Interface in"=w10914) -> ("error out"=w10912:errorcluster, "Temperature"=w10908:i8, "Interface out"=w10911:refnum<class "Interface.lvclass">)  [unwired: 7 in]
            n4609 = Greater?(x=w10908, y="Target Temp 4") -> (0:w10893:bool)
            n4610 = Select(t=w10908, s=w10893, f="Target Temp 4") -> (s? t:f=w10907:i32)
            n4611 = call-dynamic "Write Temperature.vi"("error in (no error)"=w10912, "Temperature"=w10907, "Interface in"=w10911) -> ("error out"=w10917:errorcluster, "Interface out"=w10919:refnum<class "Interface.lvclass">)  [unwired: 7 in]
            n4612 = call-dynamic "Write Interface.vi"("error in (no error)"=w10917, "Interface.lvclass"=w10919, "Channel in"=w10918) -> ("error out"=w10896:errorcluster, "Channel out"=w10897:refnum<class "Channel.lvclass">)  [unwired: 7 in]
            n4613 = case shown="True" w10893 {
              tunnel: w10896 -> [w10950 w10955]
              tunnel: w10897 -> [w10949 w10957]
              tunnel: [w10948 w10957] -> w10892
              tunnel: [w10947 w10960] -> w10889
              tunnel: w10894 -> [w10927 w10956]
              tunnel: [w10927 w10959] -> w10890
              tunnel: w10895 -> [w10926 w10952]
              tunnel: [w10926 w10958] -> w10891
              frame False {
                n4614 = call-dynamic "Read State Machine.vi"("error in (no error)"=w10950, "Device in"=w10949) -> ("error out"=w10929:errorcluster, "State Machine.lvclass"=w10936:refnum<class "State Machine.lvclass">, "Device out"=w10945:refnum<class "Channel.lvclass">)  [unwired: 7 in]
                n4615 = call-dynamic "Read ref StatesQueue.vi"("error in (no error)"=w10929, "State Machine in"=w10936) -> ("error out"=w10939:errorcluster, "ref StatesQueue"=w10933:refnum<queue>, "State Machine out"=w10935:refnum<class "State Machine.lvclass">)  [unwired: 7 in]
                n4616 = Flush Queue(queue=w10933, error in (no error)=w10939) -> (queue out=w10932:refnum<queue>, error out=w10941:errorcluster)  [unwired: 1 out]
                n4617 = Enqueue Element(queue=w10932, element=u32 35 ("State"), error in (no error)=w10941) -> (queue out=w10931:refnum<queue>, error out=w10942:errorcluster)  [unwired: 1 in, 1 out]
                n4618 = Enqueue Element(queue=w10931, element=u32 37 ("State"), error in (no error)=w10942) -> (queue out=w10930:refnum<queue>, error out=w10940:errorcluster)  [unwired: 1 in, 1 out]
                n4619 = call-dynamic "Write ref StatesQueue.vi"("error in (no error)"=w10940, "ref StatesQueue"=w10930, "State Machine in"=w10935) -> ("error out"=w10928:errorcluster, "State Machine out"=w10934:refnum<class "State Machine.lvclass">)  [unwired: 7 in]
                n4620 = call "Next State.vi"("error in (no error)"=w10928, "New_State"=u32 0, "State Machine in"=w10934) -> ("error out"=w10946:errorcluster, "State Machine out"=w10944:refnum<class "State Machine.lvclass">)  [unwired: 7 in]
                n4621 = call-dynamic "Write State Machine.vi"("error in (no error)"=w10946, "State Machine.lvclass"=w10944, "Device in"=w10945) -> ("error out"=w10947:errorcluster, "Device out"=w10948:refnum<class "Channel.lvclass">)  [unwired: 7 in]
              }
              frame True {
                # "input error"
                n4622 = call-dynamic "Read SET temp error mode.vi"("error in (no error)"=w10955, "S4GUI in"=w10956) -> ("error out"=w10954:errorcluster, "SET temp error mode"=w10951:bool, "S4GUI out"=w10953:refnum<class "S4GUI.lvclass">)  [unwired: 7 in]
                n4623 = case shown="True" w10951 {
                  tunnel: [w10969 w10982] -> w10960
                  tunnel: [w10968 w10990] -> w10959
                  tunnel: [w10964 w10989] -> w10958
                  tunnel: w10954 -> [w10963 w10982]
                  tunnel: w10953 -> [w10961 w10990]
                  tunnel: w10952 -> [w10962 w10989]
                  frame False {
                    # "last error msg"
                    n4624 = call-dynamic "Read sync.vi"("error in (no error)"=w10963, "S4ACS_GUI in"=w10961) -> ("error out"=w10965:errorcluster, "sync"=w10966:bool, "S4ACS_GUI out"=w10967:refnum<class "S4GUI.lvclass">)  [unwired: 7 in]
                    n4625 = case shown="False" w10966 {
                      tunnel: w10965 -> [w10972 w10981]
                      tunnel: [w10971 w10980] -> w10969
                      tunnel: [w10975 w10979] -> w10968
                      tunnel: w10967 -> [w10975 w10977]
                      tunnel: w10962 -> [w10973 w10976]
                      tunnel: [w10970 w10976] -> w10964
                      frame False {
                        n4626 = call-dynamic "Write Acq_state.vi"("error in (no error)"=w10972, "Acq_state"=u32 240, "Acquisition in"=w10973) -> ("error out"=w10971:errorcluster, "Acquisition out"=w10970:refnum<class "Acquisition.lvclass">)  [unwired: 7 in]
                      }
                      frame True {
                        n4627 = call-dynamic "Write Obs_state.vi"("error in (no error)"=w10981, "Obs_state"=u32 240, "S4ACS_GUI in"=w10977) -> ("error out"=w10980:errorcluster, "S4ACS_GUI out"=w10979:refnum<class "S4GUI.lvclass">)  [unwired: 7 in]
                      }
                    }
                  }
                  frame True {
                    w10984 = FALSE ("Wait Until Done")
                    # "popup msg"
                    n4628 = call <vilib>:"Application Directory.vi"() -> ("Application Directory"=w10988:path)
                    n4629 = Build Path(base path=w10988, name or relative path="MsgSetTemp.vi") -> (appended path=w10985:path)
                    n4630 = Open VI Reference(vi path=w10985) -> (vi reference=w10986:refnum<vi>, error out=w10987:errorcluster)  [unwired: 5 in]
